vi "Dynamic_eventuserdefined.vi"() -> ()   [LabVIEW 2020]
panel:
  in  "stop 2":bool
  in  "stop":bool
  out "String 2":string
  out "Boolean 2":bool
  out "Vertical Fill Slide 2":dbl
  in  "String":string
  in  "Boolean":bool
  in  "Vertical Fill Slide":dbl(slide) scale=0.0..10.0
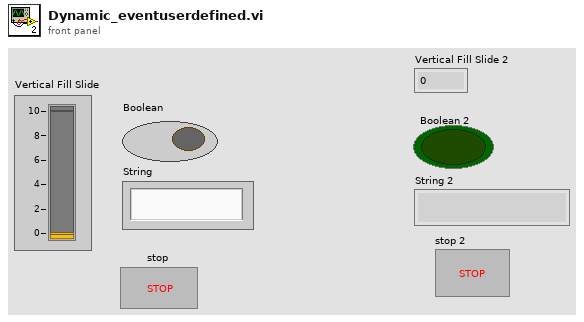
[diagram p1: front panel]
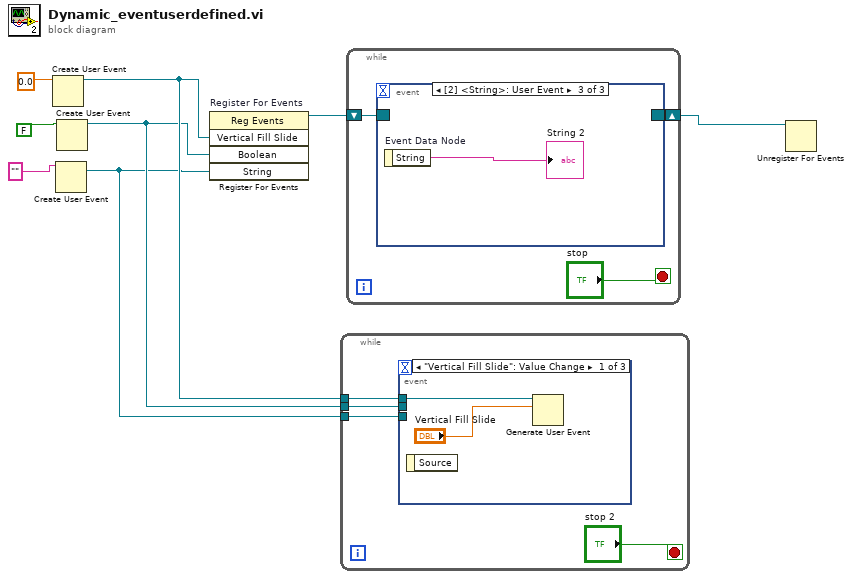
[diagram p0: block diagram]
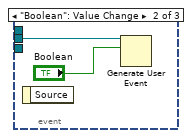
[diagram p2: hidden frame]
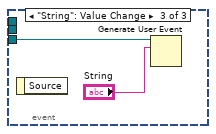
[diagram p3: hidden frame]
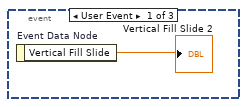
[diagram p4: hidden frame]
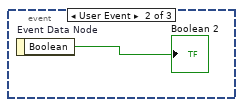
[diagram p5: hidden frame]
diagram:
  n1 = Create User Event(user event datatype=0.0 ("Vertical Fill Slide")) -> (user event=w3:refnum<user-event>)  [unwired: 1 in, 1 out]
  n2 = Create User Event(user event datatype="" ("String")) -> (user event=w1:refnum<user-event>)  [unwired: 1 in, 1 out]
  n3 = Create User Event(user event datatype=FALSE ("Boolean")) -> (user event=w2:refnum<user-event>)  [unwired: 1 in, 1 out]
  n4 = register-events "Register For Events"(w3, w2, w1) -> (reference out=w5:refnum<event-registration>)  [unwired: 2 in, 1 out]
  n5 = while {
    tunnel: w3 -> [w12]
    tunnel: w2 -> [w11]
    tunnel: w1 -> [w10]
    stop <- "stop 2" stop-if-true
    n6 = event shown="[0] \"Vertical Fill Slide\": Value Change" {
      selector: _ -> [_ _ _]
      dyn-events: _ -> [_ _ _]
      timeout: _ -> [_ _ _]
      tunnel: w12 -> [w14 _ _]
      tunnel: w11 -> [_ w16 _]
      tunnel: w10 -> [_ _ w18]
      event "Vertical Fill Slide": Value Change {
        n7 = event-data() -> ()  [unwired: 1 in, 1 out]
        n8 = Generate User Event(user event=w14, event data cluster="Vertical Fill Slide") -> ()  [unwired: 2 in, 2 out]
      }
      event "Boolean": Value Change {
        n9 = event-data() -> ()  [unwired: 1 in, 1 out]
        n10 = Generate User Event(user event=w16, event data cluster="Boolean") -> ()  [unwired: 2 in, 2 out]
      }
      event "String": Value Change {
        n11 = event-data() -> ()  [unwired: 1 in, 1 out]
        n12 = Generate User Event(user event=w18, event data cluster="String") -> ()  [unwired: 2 in, 2 out]
      }
    }
  }
  n13 = while {
    shift-right: [w20] -> w4
    shift-left: w5 -> [w21]
    stop <- "stop" stop-if-true
    n14 = event shown="[2] <String>: User Event" {
      selector: w21 -> [_ _ _]
      dyn-events: [_ _ _] -> w20
      timeout: _ -> [_ _ _]
      event User Event {
        n15 = event-data "Event Data Node"() -> ("Vertical Fill Slide"=→"Vertical Fill Slide 2":dbl)  [unwired: 1 in]
      }
      event User Event {
        n16 = event-data "Event Data Node"() -> ("Boolean"=→"Boolean 2":bool)  [unwired: 1 in]
      }
      event User Event {
        n17 = event-data "Event Data Node"() -> ("String"=→"String 2":string)  [unwired: 1 in]
      }
    }
  }
  n18 = Unregister For Events(event registration refnum=w4) -> ()  [unwired: 1 in, 1 out]
